vi "Calcul_energie.vi"(8 "Temp_en_seconde":dbl, 10 "Courant":dbl, 11 "tension":dbl) -> (2 "Energie consommé":dbl)   [LabVIEW 2019]
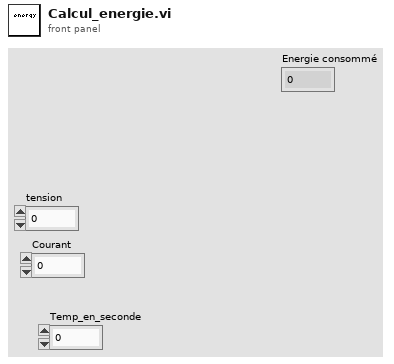
[diagram p1: front panel]
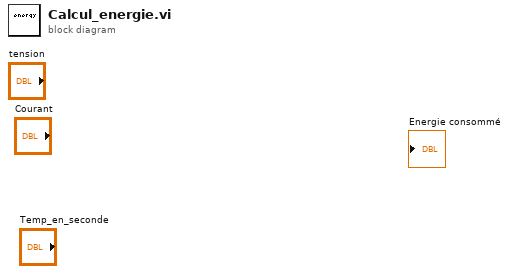
[diagram p0: block diagram]
diagram:
